vi "Delete Folder.vi"(4 "error in":errorcluster, 6 "Confirm? (T)":bool=TRUE, 7 "directory path":path=path "C:/WINDOWS/Desktop/test") -> (0 "error out":errorcluster, 2 "Deleted Folders":path[](array[path]), 3 "Deleted Files":path[](array[path]))   [LabVIEW 2011]
doc: "This example allows the user to select a parent directory and delete that directory, all of its subdirectories, and all of the files contained within those folders. Currently, the delete function in the File I/O->Advanced Palette will only delete a directory when it is completely empty. \n\nThis example drills down into the folder as far as it can go and then deletes that folder and all of it's contents. It uses shift registers to change the directory path for each iteration of the loop. It then works its way up the tree deleting each folder until it reaches and deletes the parent folder."
panel:
  # "See File->VI Properties->Documentation for a description of this VI."
  # "WARNING: This example deletes all of the contents from the folder\nthat you specify in the directory path control above. Make sure you \ndo not select a folder that contains important documents or subfolders."
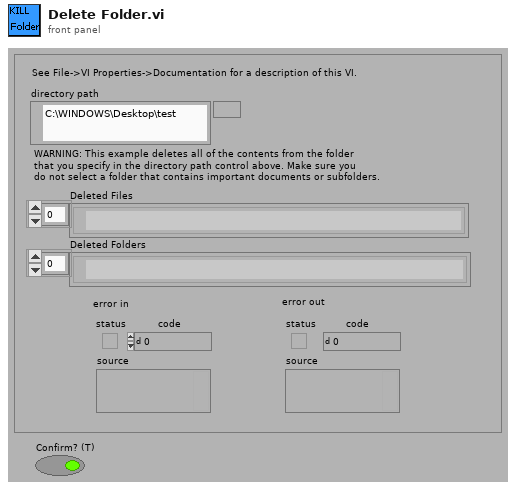
[diagram p1: front panel]
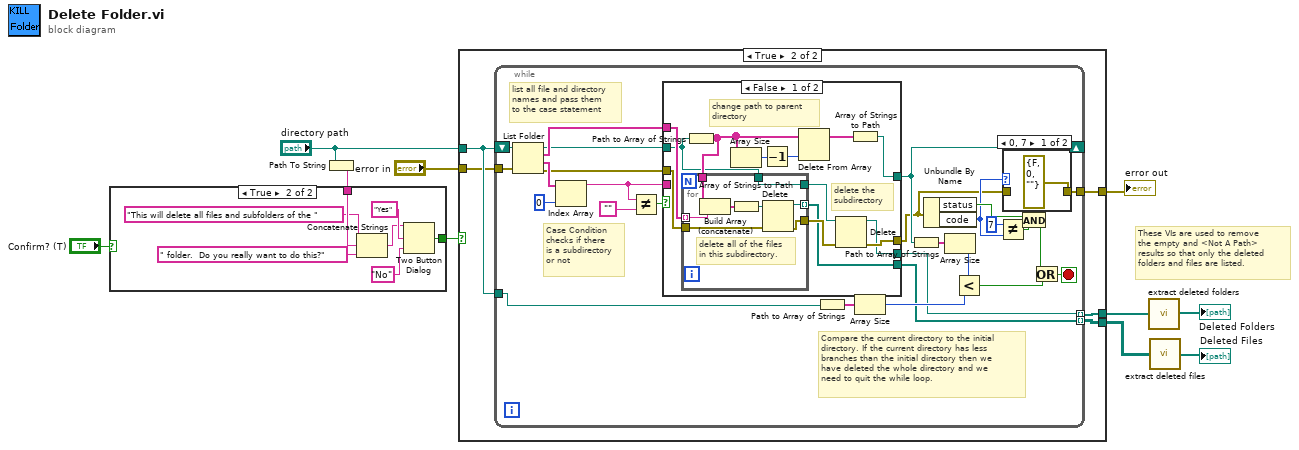
[diagram p0: block diagram]
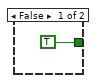
[diagram p2: hidden frame]
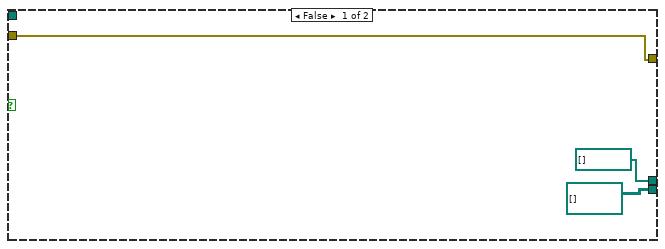
[diagram p3: hidden frame]
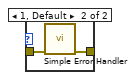
[diagram p4: hidden frame]
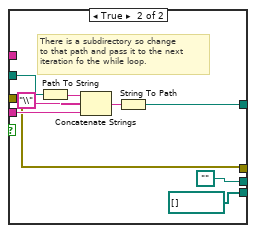
[diagram p5: hidden frame]
diagram:
  # "These VIs are used to remove \nthe empty and <Not A Path> \nresults so that only the deleted \nfolders and files are listed."
  n1 = Path To String(path="directory path") -> (string=w8:string)
  n2 = case shown="True" "Confirm? (T)" {
    tunnel: [TRUE ("T button?") w18] -> w10
    tunnel: w8 -> [_ w17]
    frame False {
    }
    frame True {
      n3 = Concatenate Strings("This will delete all files and subfolders of the " ("message"), w17, " folder.  Do you really want to do this?" ("Substring")) -> (w12:string)
      n4 = Two Button Dialog(message=w12, 1:"No" ("F button name (\"Cancel\")"), 2:"Yes" ("T button name (\"OK\")")) -> (T button?=w18:bool)
    }
  }
  n5 = case shown="True" w10 {
    tunnel: "directory path" -> [_ w26]
    tunnel: "error in" -> [w21 w25]
    tunnel: [w21 w24] -> w6
    tunnel: [path[][] [] w23] -> w3
    tunnel: [path[] [] w22] -> w5
    frame False {
    }
    frame True {
      n6 = while {
        tunnel: [w28] -> w22 mode=indexing
        tunnel: [w29] -> w23 mode=indexing
        tunnel: [w30] -> w24
        tunnel: w25 -> [w31]
        tunnel: w26 -> [w27]
        shift-left: w26 -> [w51]
        shift-right: [w45] -> _
        stop <- w38 stop-if-true
        # "Compare the current directory to the initial\ndirectory. If the current directory has less \nbranches than the initial directory then we\nhave deleted the whole directory and we \nneed to quit the while loop."
        # "Case Condition\nchecks if there\nis a subdirectory\nor not"
        # "list all file and directory\nnames and pass them \nto the case statement"
        n7 = List Folder(path=w51, error in=w31) -> (path out=w46:path, filenames=w52:string[], folder names=w53:string[], error out=w39:errorcluster)  [unwired: 2 out]
        n8 = Index Array(array=w53, index=0 ("Index")) -> (element=w49:string)
        n9 = Not Equal?(x=w49, y="") -> (x != y?=w47:bool)
        n10 = case shown="False" w47 {
          tunnel: w49 -> [_ w83]
          tunnel: [w66 w85] -> w45
          tunnel: w46 -> [w63 w82]
          tunnel: w52 -> [w65 _]
          tunnel: w39 -> [w61 w80]
          tunnel: [w59 w80] -> w32
          tunnel: [w57 path[] []] -> w29
          tunnel: [w58 path "" ("dup path")] -> w28
          frame False {
            # "change path to parent\ndirectory"
            # "delete the \nsubdirectory"
            n11 = Path to Array of Strings(0:w63) -> (2:w64:string[])  [unwired: 1 out]
            n12 = for {
              tunnel: w65 -> [w75] mode=indexing
              tunnel: w64 -> [w77]
              tunnel: w63 -> [w76]
              tunnel: [w76] -> w62
              tunnel: w61 -> [w72]
              tunnel: [w71] -> w60
              tunnel: [w70] -> w57 mode=indexing
              # "delete all of the files\nin this subdirectory."
              n13 = Build Array (concatenate)(w77, w75) -> (w74:string[])
              n14 = Array of Strings to Path(0:w74) -> (2:w73:path)  [unwired: 1 out]
              n15 = Delete(path (use dialog)=w73, error in=w72) -> (deleted path=w70:path, error out=w71:errorcluster)  [unwired: 4 out]
            }
            n16 = Array Size(array=w64) -> (size(s)=w69:i32)
            n17 = Decrement(x=w69) -> (x-1=w68:i32)
            n18 = Delete From Array(array=w64, index=w68) -> (array with subset deleted=w67:string[])  [unwired: 1 in, 1 out]
            n19 = Delete(path (use dialog)=w62, error in=w60) -> (deleted path=w58:path, error out=w59:errorcluster)  [unwired: 4 out]
            n20 = Array of Strings to Path(0:w67) -> (2:w66:path)  [unwired: 1 out]
          }
          frame True {
            # "There is a subdirectory so change\nto that path and pass it to the next\niteration fo the while loop."
            n21 = Path To String(path=w82) -> (string=w81:string)
            n22 = Concatenate Strings(w81, "\\", w83) -> (w86:string)
            n23 = String To Path(string=w86) -> (path=w85:path)
          }
        }
        n24 = Path to Array of Strings(0:w27) -> (2:w43:string[])  [unwired: 1 out]
        n25 = Array Size(array=w43) -> (size(s)=w41:i32)
        n26 = Path to Array of Strings(0:w45) -> (2:w44:string[])  [unwired: 1 out]
        n27 = Unbundle By Name(w32) -> ("status"=w37:bool, "code"=w33:i32)
        n28 = Array Size(array=w44) -> (size(s)=w42:i32)
        n29 = Less?(x=w42, y=w41) -> (x < y?=w40:bool)
        n30 = Not Equal?(x=7, y=w33) -> (x != y?=w36:bool)
        n31 = case shown="0, 7" w33 {
          tunnel: w32 -> [_ w56]
          tunnel: [errorcluster {"status"=FALSE, "code"=0, "source"=""} ("error out") w55] -> w30
          frame 0, 7 {
          }
          frame 1, Default {
            n32 = call <vilib>:"Simple Error Handler.vi"("error in (no error)"=w56) -> ("error out"=w55:errorcluster)  [unwired: 1 in, 7 out]
          }
        }
        n33 = And(x=w37, y=w36) -> (x .and. y?=w35:bool)
        n34 = Or(x=w35, y=w40) -> (x .or. y?=w38:bool)
      }
    }
  }
  "error out" <- w6
  n35 = call "extract deleted folders.vi"("Input Array"=w5) -> ("Deleted Folders"=→"Deleted Folders":path[])
  n36 = call "extract deleted files.vi"("Input Array"=w3) -> ("Deleted Files"=→"Deleted Files":path[])
